vi "HGF_TaskDFSM.appendData2Variant.vi"(0 "initData":variant, 1 "deviceFactory":refnum<class "HGF_Factory.lvclass">, 2 "autoConfigVisitor":refnum<class "HGF_DeviceVisitor.lvclass">, 3 "autoConfigure":bool, 4 "statusPublisher":refnum<class "HGF_PVPublisher.lvclass">, 5 "error in (no error)":errorcluster) -> (14 "dup initData":variant, 19 "error out":errorcluster)   [LabVIEW 2012, in "HGF_DeviceFSM.lvlib" / "HGF_TaskDFSM.lvclass"]
uses:
  HGF_TaskDFSM.lvclass
  HGF_DeviceBaseClasses/HGF_DeviceVisitor/HGF_DeviceVisitor.lvclass
  HGF_BaseClasses/HGF_PVPublisher/HGF_PVPublisher.lvclass
  HGF_BaseClasses/HGF_Factory/HGF_Factory.lvclass
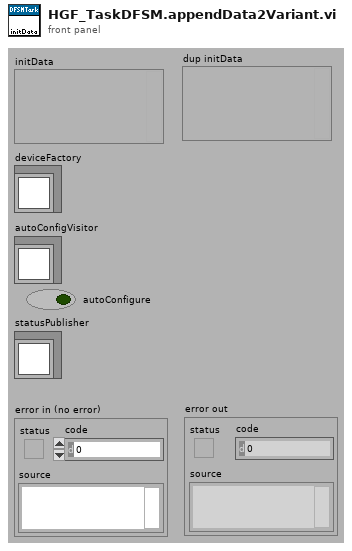
[diagram p1: front panel]
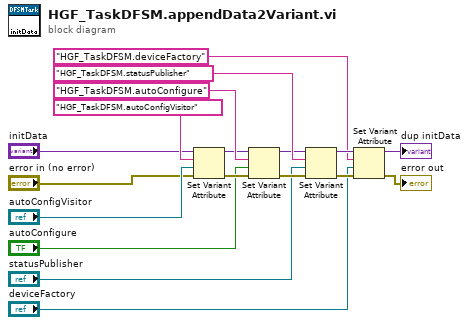
[diagram p0: block diagram]
diagram:
  n1 = Set Variant Attribute(Variant="initData", name="HGF_TaskDFSM.autoConfigVisitor", value="autoConfigVisitor", error in="error in (no error)") -> (Variant out=w12:variant, error out=w15:errorcluster)  [unwired: 1 out]
  n2 = Set Variant Attribute(Variant=w12, name="HGF_TaskDFSM.autoConfigure", value="autoConfigure", error in=w15) -> (Variant out=w13:variant, error out=w14:errorcluster)  [unwired: 1 out]
  n3 = Set Variant Attribute(Variant=w13, name="HGF_TaskDFSM.statusPublisher", value="statusPublisher", error in=w14) -> (Variant out=w5:variant, error out=w6:errorcluster)  [unwired: 1 out]
  n4 = Set Variant Attribute(Variant=w5, name="HGF_TaskDFSM.deviceFactory", value="deviceFactory", error in=w6) -> (Variant out=→"dup initData":variant, error out=→"error out":errorcluster)  [unwired: 1 out]
